vi "_ProcessCalData.vi"(6 "CalResultIn":T1[](array[typedef]), 8 "Resolution":dbl[][](array[numeric]) format="%.2f", 9 "Calibration":dbl[][](array[numeric]) format="%.2f", 10 "MassReference":cluster{"Mass":dbl, "Use":bool}[](array[cluster]), 11 "PeakSearchParameters":dbl[](array[numeric])) -> (0 "ResolutionOut":dbl[][](array[numeric]) format="%.2f", 1 "CalibrationOut":dbl[][](array[numeric]) format="%.2f", 2 "ResOK":bool, 3 "CalOK":bool, 4 "AllFound":bool, 5 "CalResultOut":T1[](array[typedef]), 7 "AllValid":bool)   [LabVIEW 2015]
uses:
  Type/_CalibrationResult.ctl
  Type/_Data Operation.ctl
  Type/_Log Command.ctl
panel:
  # "MinimumMassPeakWidth"
  # "ThresholdForMassSpectrum"
  # "SearchRange"
  # "NumberOfSmooth"
  # "NumberOfPointsToSmooth"
  # "WidthAtOfMaximum"
  # "PeakFindingNoiseLevel"
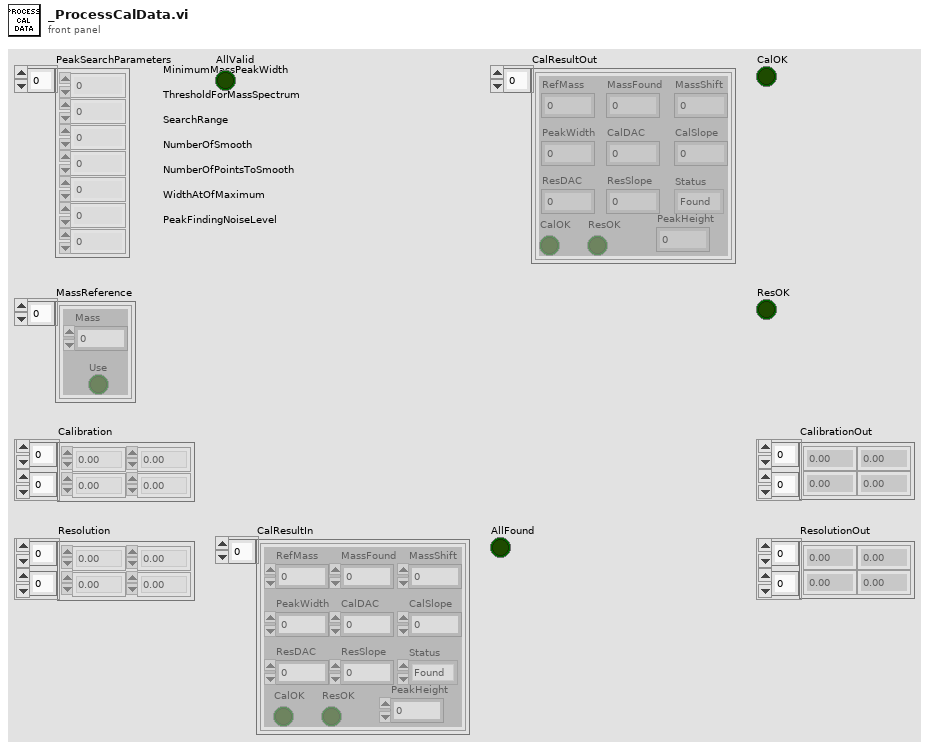
[diagram p1: front panel]
types:
  T1 = typedef "_CalibrationResult.ctl" = cluster{"RefMass":dbl, "MassFound":dbl, "MassShift":dbl, "PeakWidth":dbl, "CalDAC":dbl, "CalSlope":dbl, "ResDAC":dbl, "ResSlope":dbl, "Status":enum16{"Found", "Missing", "Not Used"}, "CalOK":bool, "ResOK":bool, "PeakHeight":dbl}
  T2 = typedef "_Log Command.ctl" = enum16{"No Command", "Open", "Read", "Write", "Close", "Check Size"}
  T3 = typedef "_Data Operation.ctl" = enum8{"Initialize", "Get Data", "Set Data", "Close"}
  T4 = typedef "_Current Data.ctl" = cluster{"Scan#":i32, "Run Time (mS)":i32, "TIC X":dbl[], "TIC Y":dbl[][], "MassRange":cluster{"X Title":string, "X":dbl[], "Y":i32[]}[], "Fixed Mass (amu)":dbl, "Method":T5}
  T5 = typedef "_XML Expt.ctl" = cluster{"StartT(mS)":i32, "#Cycles":i32, "PauseT(uS)":i32, "ScanType":i32, "Polarity":u8, "FixedMass":dbl, "DelayT(mS)":i32, "Active Ch":T6[], "Mass Range":T7[]}
  T6 = typedef "_XML Lens.ctl" = cluster{"Value":dbl, "ChID":u8}
  T7 = typedef "_Mass Range Property.ctl" = cluster{"Start":dbl, "Stop":dbl, "Step Size":dbl, "Steps":i32, "Dwell":dbl, "Parameters":T8[], "Res":T9}
  T8 = typedef "_Mass Range Parameters.ctl" = cluster{"Name":string, "Ch#":u8, "StartV":dbl, "StopV":dbl, "StepV":dbl, "Index":u8}
  T9 = typedef "_RT Res Type.ctl" = u16
  T10 = typedef "_Peak Property.ctl" = cluster{"Centroid":dbl, "Height":dbl, "FWHM":dbl, "Resolution":dbl, "Area":dbl, "StoN":dbl, "ApexX":dbl, "Baseline":dbl, "LEdgeX":dbl, "LEdgeY":dbl, "REdgeX":dbl, "REdgeY":dbl, "LEdgeFWHM":dbl, "REdgeFWHM":dbl}
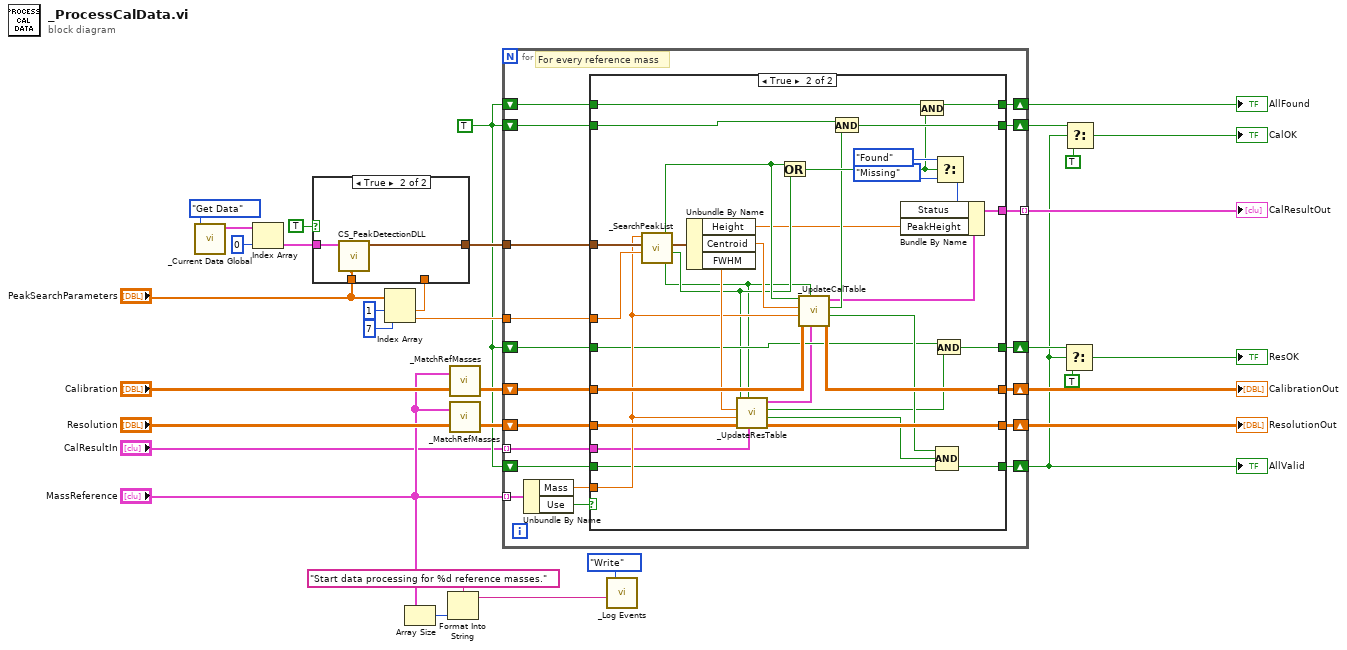
[diagram p0: block diagram]
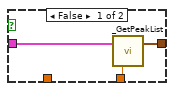
[diagram p2: hidden frame]
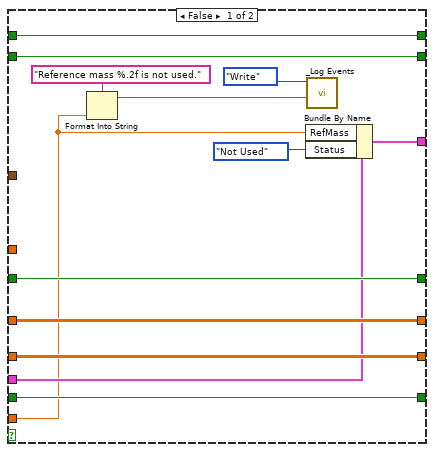
[diagram p3: hidden frame]
diagram:
  w12 = TRUE
  n1 = call "_Current Data Global.vi"("Operation"=_Data_Operation."Get Data") -> ("CurrentData"=w32:T4[])  [unwired: 3 in, 3 out]
  n2 = Index Array(array=w32, index=0) -> (element=w19:T4)
  n3 = Index Array(array="PeakSearchParameters", index #1=1 ("index"), index #2=7 ("index")) -> (element #1=w29:dbl, element #2=w27:dbl)
  n4 = case shown="True" TRUE {
    tunnel: w29 -> [w36 _]
    tunnel: [w35 w38] -> w28
    tunnel: w19 -> [w34 w39]
    tunnel: "PeakSearchParameters" -> [_ w37]
    frame False {
      n5 = call "_GetPeakList.vi"("Minimum Height (100)"=w36, "Current Data"=w34) -> ("PeakList"=w35:T10[])  [unwired: 1 in]
    }
    frame True {
      n6 = call "CS_PeakDetectionDLL.vi"("PeakSearchParameters"=w37, "Current Data"=w39) -> ("Peak List"=w38:T10[])  [unwired: 8 in, 1 out]
    }
  }
  n7 = Array Size(array="MassReference") -> (size(s)=w23:i32)
  n8 = Format Into String(format string="Start data processing for %d reference masses.", w23) -> (resulting string=w20:string)  [unwired: 2 in, 1 out]
  n9 = call "_MatchRefMasses.vi"("Cal/Res Table"="Calibration", "MassReference"="MassReference") -> ("Cal/Res Table Out"=w16:dbl[][])  [unwired: 1 in]
  n10 = call "_MatchRefMasses.vi"("Cal/Res Table"="Resolution", "MassReference"="MassReference") -> ("Cal/Res Table Out"=w15:dbl[][])  [unwired: 1 in]
  n11 = for {
    tunnel: "MassReference" -> [w58] mode=indexing
    tunnel: w28 -> [w55]
    tunnel: "CalResultIn" -> [w41] mode=indexing
    tunnel: w27 -> [w54]
    tunnel: [w40] -> w26 mode=indexing
    shift-right: [w52] -> w8
    shift-left: w12 -> [w53]
    shift-right: [w50] -> w11
    shift-left: w12 -> [w51]
    shift-right: [w48] -> w25
    shift-left: w16 -> [w49]
    shift-right: [w46] -> w24
    shift-left: w15 -> [w47]
    shift-right: [w44] -> w18
    shift-left: w12 -> [w45]
    shift-right: [w42] -> w7
    shift-left: w12 -> [w43]
    # "For every reference mass"
    n12 = Unbundle By Name(w58) -> ("Mass"=w56:dbl, "Use"=w57:bool)
    n13 = case shown="True" w57 {
      tunnel: w56 -> [w61 w91]
      tunnel: w55 -> [_ w105]
      tunnel: w54 -> [_ w104]
      tunnel: w53 -> [w71 w100]
      tunnel: [w71 w99] -> w52
      tunnel: w51 -> [w70 w79]
      tunnel: [w70 w80] -> w50
      tunnel: w49 -> [w69 w98]
      tunnel: [w69 w97] -> w48
      tunnel: w47 -> [w68 w96]
      tunnel: [w68 w95] -> w46
      tunnel: w45 -> [w64 w93]
      tunnel: [w64 w92] -> w44
      tunnel: [w63 w88] -> w42
      tunnel: w43 -> [w63 w89]
      tunnel: w41 -> [w62 w83]
      tunnel: [w59 w74] -> w40
      frame False {
        n14 = Format Into String(format string="Reference mass %.2f is not used.", w61) -> (resulting string=w65:string)  [unwired: 2 in, 1 out]
        n15 = Bundle By Name(cluster=w62, "RefMass"=w61, "Status"=enum16{"Found", "Missing", "Not Used"}."Not Used") -> (w59:T1)
        n16 = call "_Log Events.vi"("Event"=w65, "Log Command"=_Log_Command."Write") -> ()  [unwired: 6 in, 2 out]
      }
      frame True {
        n17 = call "_SearchPeakList.vi"("Search Window (3)"=w104, "Peak List"=w105, "RefMass"=w91) -> ("Valid Peak?"=w72:bool, "Found 2"=w77:bool, "Peak"=w103:T10, "Found"=w86:bool)  [unwired: 1 in]
        n18 = Unbundle By Name(w103) -> ("Height"=w73:dbl, "Centroid"=w90:dbl, "FWHM"=w94:dbl)
        n19 = call "_UpdateResTable.vi"("CalResultIn"=w83, "Valid Peak?"=w72, "Resolution"=w96, "RefMass"=w91, "FoundPW"=w94, "Found"=w77) -> ("ResolutionOut"=w95:dbl[][], "ResValid"=w82:bool, "ResOK"=w81:bool, "CalResultOut"=w78:T1)  [unwired: 2 out]
        n20 = Or(x=w86, y=w77) -> (x .or. y?=w87:bool)
        n21 = call "_UpdateCalTable.vi"("CalResultIn"=w78, "Valid Peak?"=w72, "Calibration"=w98, "RefMass"=w91, "MassFound"=w90, "Found"=w86) -> ("CalibrationOut"=w97:dbl[][], "CalValid"=w85:bool, "CalOK"=w84:bool, "CalResultOut"=w76:T1)  [unwired: 2 out]
        n22 = And(x=w100, y=w84) -> (x .and. y?=w99:bool)
        n23 = And(x=w93, y=w87) -> (x .and. y?=w92:bool)
        n24 = And(x=w79, y=w81) -> (x .and. y?=w80:bool)
        n25 = Select(t=enum16{"Found", "Missing", "Not Used"}."Found" ("Status"), s=w87, f=enum16{"Found", "Missing", "Not Used"}."Missing" ("Status")) -> (s? t:f=w75:enum16{"Found", "Missing", "Not Used"})
        n26 = Bundle By Name(cluster=w76, "Status"=w75, "PeakHeight"=w73) -> (w74:T1)
        n27 = Compound Arithmetic op=AND(w85, w82, w89) -> (w88:bool)
      }
    }
  }
  "CalResultOut" <- w26
  "CalibrationOut" <- w25
  "ResolutionOut" <- w24
  "AllFound" <- w18
  "AllValid" <- w7
  n28 = call "_Log Events.vi"("Event"=w20, "Log Command"=_Log_Command."Write") -> ()  [unwired: 6 in, 2 out]
  n29 = Select(t=w11, s=w7, f=TRUE) -> (s? t:f=→"ResOK":bool)
  n30 = Select(t=w8, s=w7, f=TRUE) -> (s? t:f=→"CalOK":bool)
